vi "Run.vi"(8 "error in (no error)":errorcluster, 11 "Terminal Menus in":refnum<class "Terminal Menus.lvclass">) -> (0 "error out":errorcluster, 3 "Terminal Menus out":refnum<class "Terminal Menus.lvclass">)   [LabVIEW 2016, in "CLD Exam - ATM.lvlib" / "Terminal Menus.lvclass"]
uses:
  Terminal Menus.lvclass
  D:/Repos/Stream/software/Mediator/Classes/Mediated Actor/Mediated Actor.lvclass
  Mediator/Classes/Message Interface/Message Interface.lvclass
  Terminal Menus.lvclass/Terminal Menus.ctl
  Log/Application Log/Log Level.ctl
  Mediator/Classes/Message String/Message String.lvclass
  Mediator/Classes/Mediated Actor/Mediated Actor.lvclass
  Log/Application Log/Application Log.lvclass
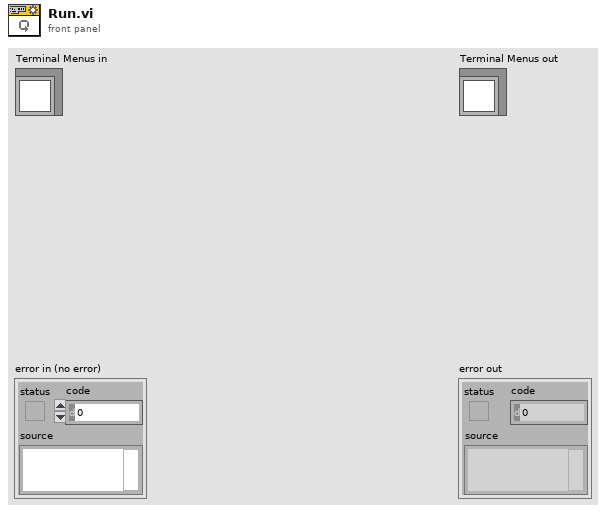
[diagram p1: front panel]
types:
  T1 = cluster{"Account Action Completed":refnum<event-registration>, "System Exit":refnum<event-registration>, "To Self":refnum<event-registration>}
  T2 = typedef "Stream Log.lvlib/Application Log.lvclass/Log Level.ctl" = enum16{"Imperative", "Major", "Minor", "Debug", "Off"}
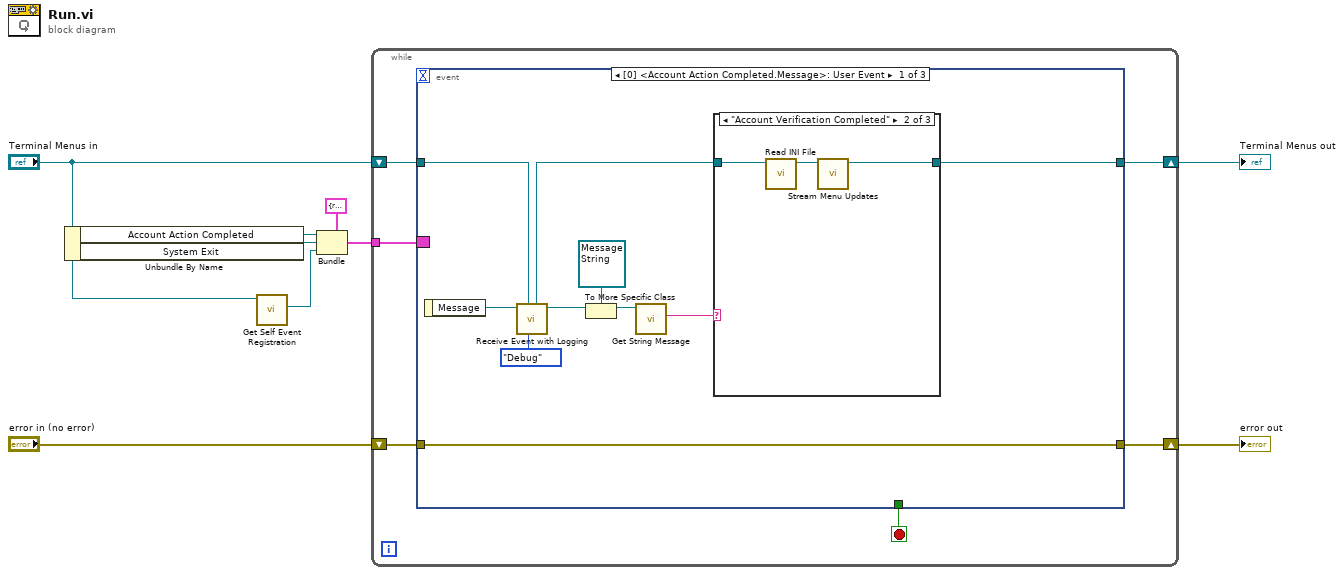
[diagram p0: block diagram]
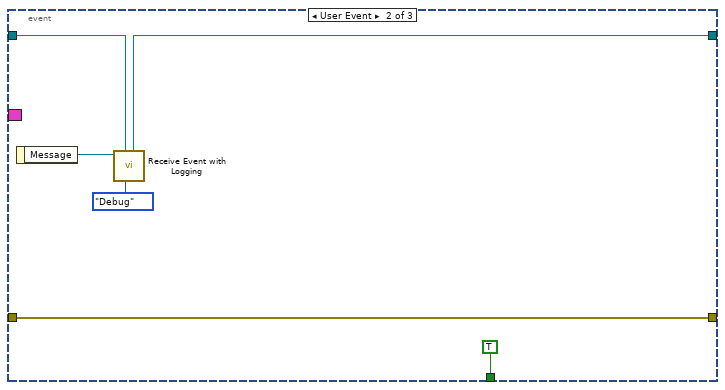
[diagram p4: hidden frame]
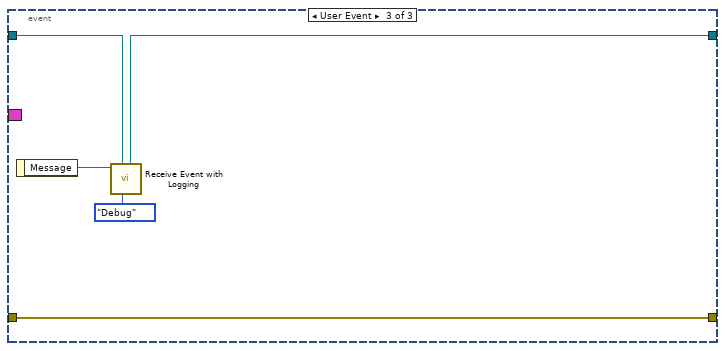
[diagram p5: hidden frame]
diagram:
  n1 = Unbundle By Name("Terminal Menus in") -> ("Account Action Completed"=w6:refnum<event-registration>, "System Exit"=w5:refnum<event-registration>)
  n2 = call "Get Self Event Registration.vi"("Mediated Actor in"="Terminal Menus in") -> ("Event Registration Refnum"=w2:refnum<event-registration>)  [unwired: 9 in, 1 out]
  n3 = Bundle(cluster=T1 {"Account Action Completed"=refnum, "System Exit"=refnum, "To Self"=refnum}, "Account Action Completed"=w6, "System Exit"=w5, "To Self"=w2) -> (w3:T1)
  n4 = while {
    shift-right: [w14] -> w9
    shift-left: "Terminal Menus in" -> [w15]
    shift-right: [w12] -> w7
    shift-left: "error in (no error)" -> [w13]
    tunnel: w3 -> [w11]
    stop <- w10 stop-if-true
    n5 = event shown="[0] <Account Action Completed.Message>: User Event" {
      selector: w11 -> [_ _ _]
      dyn-events: _ -> [_ _ _]
      timeout: _ -> [_ _ _]
      tunnel: w15 -> [w22 w33 w39]
      tunnel: [w24 w32 w38] -> w14
      tunnel: w13 -> [w25 w36 w41]
      tunnel: [w25 w36 w41] -> w12
      tunnel: [_ TRUE _] -> w10
      event User Event {
        n6 = event-data() -> ("Message"=w23:refnum<class "Message Interface.lvclass">)  [unwired: 1 in]
        n7 = call "Receive Event with Logging.vi"("Global Log Level"=Log_Level."Debug", "Mediated Actor in"=w22, "Message"=w23) -> ("Message out"=w19:refnum<class "Message Interface.lvclass">, "Mediated Actor out"=w21:refnum<class "Terminal Menus.lvclass">)  [unwired: 5 in, 2 out]
        n8 = To More Specific Class(target class=refnum<class "Message String.lvclass"> refnum ("Message String in"), reference=w19) -> (specific class reference=w18:refnum<class "Message String.lvclass">)  [unwired: 1 in, 1 out]
        n9 = call "Get String Message.vi"("Message String in"=w18) -> ("Name"=w16:string)  [unwired: 7 in, 3 out]
        n10 = case shown="\"Account Verification Completed\"" w16 {
          tunnel: [w26 w28 w30] -> w24
          tunnel: w21 -> [w26 w27 w30]
          frame "Failed" {
          }
          frame "Account Verification Completed" {
            n11 = call "Read INI File.vi"("Terminal Menus in"=w27) -> ("Terminal Menus out"=w29:refnum<class "Terminal Menus.lvclass">)  [unwired: 9 in, 1 out]
            n12 = call "Stream Menu Updates.vi"("Terminal Menus in"=w29) -> ("Terminal Menus out"=w28:refnum<class "Terminal Menus.lvclass">)  [unwired: 9 in, 1 out]
          }
          frame Default {
          }
        }
      }
      event User Event {
        n13 = event-data() -> ("Message"=w34:refnum<class "Message Interface.lvclass">)  [unwired: 1 in]
        n14 = call "Receive Event with Logging.vi"("Global Log Level"=Log_Level."Debug", "Mediated Actor in"=w33, "Message"=w34) -> ("Mediated Actor out"=w32:refnum<class "Terminal Menus.lvclass">)  [unwired: 5 in, 3 out]
      }
      event User Event {
        n15 = event-data() -> ("Message"=w40:refnum<class "Message Interface.lvclass">)  [unwired: 1 in]
        n16 = call "Receive Event with Logging.vi"("Global Log Level"=Log_Level."Debug", "Mediated Actor in"=w39, "Message"=w40) -> ("Mediated Actor out"=w38:refnum<class "Terminal Menus.lvclass">)  [unwired: 5 in, 3 out]
      }
    }
  }
  "error out" <- w7
  "Terminal Menus out" <- w9
